vi "Get Bind Address.vi"(8 "error in (no error)":errorcluster, 11 "Node in":refnum<class "Node.lvclass">) -> (0 "error out":errorcluster, 2 "Bind Address":string, 3 "Node out":refnum<class "Node.lvclass">)   [LabVIEW 2020, in "VolatusConfig.lvlib" / "Node.lvclass"]
uses:
  Node.lvclass
  Node.lvclass/Node.ctl
  VolatusConfigElement/VolatusConfigElement.lvclass
  lv-cdm/CDM-Config/Config Element/Config Element.lvclass
  C:/dev/lv20CE/relink/lv-volatus/VolatusConfig/VolatusConfigElement/VolatusConfigElement.lvclass
  C:/dev/lv20CE/relink/lv-volatus/VolatusConfig/Node/Node.lvclass
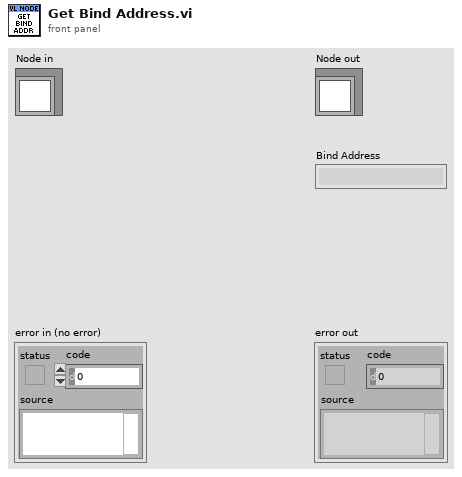
[diagram p1: front panel]
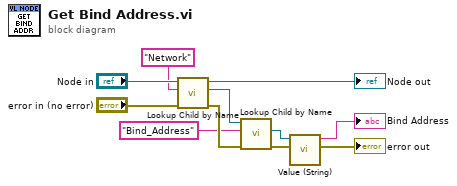
[diagram p0: block diagram]
diagram:
  n1 = call "Lookup Child by Name.vi"("error in (no error)"="error in (no error)", "Child Name"="Network", "VolatusConfigElement in"="Node in") -> ("error out"=w6:errorcluster, "Child"=w7:refnum<class "Config Element.lvclass">, "VolatusConfigElement out"=→"Node out":refnum<class "Node.lvclass">)  [unwired: 5 in, 1 out]
  n2 = call "Lookup Child by Name.vi"("error in (no error)"=w6, "Name"="Bind_Address", "Config Element in"=w7) -> ("error out"=w4:errorcluster, "Child"=w3:refnum<class "Config Element.lvclass">)  [unwired: 5 in, 2 out]
  n3 = call "Value (String).vi"("error in (no error)"=w4, "Config Element in"=w3) -> ("error out"=→"error out":errorcluster, "String Value"=→"Bind Address":string)  [unwired: 8 in]
